vi "CountsToTheta.vi"(10 "Link2EncPos":dbl, 11 "Link1EncPos":dbl) -> (2 "Theta1":dbl, 3 "Theta0":dbl)   [LabVIEW 2017, in "controllerLibrary.lvlib"]
uses:
  controllerLibrary.lvlib
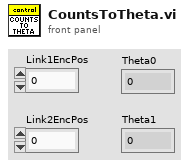
[diagram p1: front panel]
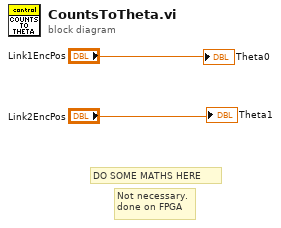
[diagram p0: block diagram]
diagram:
  # "Not necessary.\ndone on FPGA"
  # "DO SOME MATHS HERE"
  "Theta1" <- "Link2EncPos"
  "Theta0" <- "Link1EncPos"
